vi "nanocal -- nuclear schottky fit -- 2x2 -- V9.vi"() -> ()   [LabVIEW 2021] (continued)
\"κ0\" -> 0.000000000000   ,  \"mm1\" -> 0.000000000000   ,  \"mm2\" -> 0.000000000000   ,  \"mm3\" -> 0.000000000000   ,  \"T\" -> 1.120000000000   ,  \"B\" -> 10.000000000000   ,  \"θ\" -> 0.000000000000   ,  \"Reoff\" -> 0.000000000000   ,  \"Imoff\" -> 0.000000000000   ,  \"στ1\" -> 0.000000000000   ,  \"στS\" -> 0.000000000000   ,  \"στN\" -> 0.000000000000    |>   , \n\"IDS0436_220527_RAW_cal__ref_\" ->   <|    \"ζ\" -> 0.020634042480   ,  \"τ1\" -> 0.020416898580   ,  \"τS\" -> 0.013006754143   ,  \"τN\" -> 0.000157221748   ,  \"τC\" -> 0.001868338850   ,  \"κ0\" -> 0.000000012250   ,  \"mm1\" -> 0.000033184482   ,  \"mm2\" -> 0.014698009084   ,  \"mm3\" -> 0.020989645793   ,  \"T\" -> 1.900000000000   ,  \"B\" -> 10.000000000000   ,  \"θ\" -> 0.000000000000   ,  \"Reoff\" -> -693877.551020413636   ,  \"Imoff\" -> 0.000000000000   ,  \"στ1\" -> 0.001009802597   ,  \"στS\" -> 0.000108538250   ,  \"στN\" -> 0.000005592624    |>   , \n\"IDS0436_220527_RAW_cal__sam_\" ->   <|    \"ζ\" -> 0.000000000000   ,  \"τ1\" -> 0.000000000000   ,  \"τS\" -> 0.000000000000   ,  \"τN\" -> 0.000000000000   ,  \"τC\" -> 0.000000000000   ,  \"κ0\" -> 0.000000000000   ,  \"mm1\" -> 0.000000000000   ,  \"mm2\" -> 0.000000000000   ,  \"mm3\" -> 0.000000000000   ,  \"T\" -> 1.900000000000   ,  \"B\" -> 10.000000000000   ,  \"θ\" -> 0.000000000000   ,  \"Reoff\" -> 0.000000000000   ,  \"Imoff\" -> 0.000000000000   ,  \"στ1\" -> 0.000000000000   ,  \"στS\" -> 0.000000000000   ,  \"στN\" -> 0.000000000000    |>   , \n\"IDS0437_220527_RAW_cal__ref_\" ->   <|    \"ζ\" -> 0.017700486500   ,  \"τ1\" -> 0.021195716861   ,  \"τS\" -> 0.009553240691   ,  \"τN\" -> 0.000096318625   ,  \"τC\" -> 0.001777778444   ,  \"κ0\" -> 0.000000022000   ,  \"mm1\" -> 0.000026199986   ,  \"mm2\" -> 0.011360732885   ,  \"mm3\" -> 0.021406923644   ,  \"T\" -> 3.100000000000   ,  \"B\" -> 10.000000000000   ,  \"θ\" -> 0.000000000000   ,  \"Reoff\" -> -326530.612244898453   ,  \"Imoff\" -> 0.000000000000   ,  \"στ1\" -> 0.003823035587   ,  \"στS\" -> 0.000080670014   ,  \"στN\" -> 0.000008312416    |>   , \n\"IDS0437_220527_RAW_cal__sam_\" ->   <|    \"ζ\" -> 0.000000000000   ,  \"τ1\" -> 0.000000000000   ,  \"τS\" -> 0.000000000000   ,  \"τN\" -> 0.000000000000   ,  \"τC\" -> 0.000000000000   ,  \"κ0\" -> 0.000000000000   ,  \"mm1\" -> 0.000000000000   ,  \"mm2\" -> 0.000000000000   ,  \"mm3\" -> 0.000000000000   ,  \"T\" -> 3.100000000000   ,  \"B\" -> 10.000000000000   ,  \"θ\" -> 0.000000000000   ,  \"Reoff\" -> 0.000000000000   ,  \"Imoff\" -> 0.000000000000   ,  \"στ1\" -> 0.000000000000   ,  \"στS\" -> 0.000000000000   ,  \"στN\" -> 0.000000000000    |>   , \n\"IDS0438_220527_RAW_cal__ref_\" ->   <|    \"ζ\" -> 0.017333863476   ,  \"τ1\" -> 0.021487771905   ,  \"τS\" -> 0.006060943357   ,  \"τN\" -> 0.000094743973   ,  \"τC\" -> 0.001680463551   ,  \"κ0\" -> 0.000000054800   ,  \"mm1\" -> 0.000022565233   ,  \"mm2\" -> 0.007769356044   ,  \"mm3\" -> 0.021638703353   ,  \"T\" -> 5.700000000000   ,  \"B\" -> 10.000000000000   ,  \"θ\" -> 0.000000000000   ,  \"Reoff\" -> -102040.816326530650   ,  \"Imoff\" -> 0.000000000000   ,  \"στ1\" -> 0.003634760564   ,  \"στS\" -> 0.000066823566   ,  \"στN\" -> 0.000004946508    |>   , \n\"IDS0438_220527_RAW_cal__sam_\" ->   <|    \"ζ\" -> 0.000000000000   ,  \"τ1\" -> 0.000000000000   ,  \"τS\" -> 0.000000000000   ,  \"τN\" -> 0.000000000000   ,  \"τC\" -> 0.000000000000   ,  \"κ0\" -> 0.000000000000   ,  \"mm1\" -> 0.000000000000   ,  \"mm2\" -> 0.000000000000   ,  \"mm3\" -> 0.000000000000   ,  \"T\" -> 5.700000000000   ,  \"B\" -> 10.000000000000   ,  \"θ\" -> 0.000000000000   ,  \"Reoff\" -> 0.000000000000   ,  \"Imoff\" -> 0.000000000000   ,  \"στ1\" -> 0.000000000000   ,  \"στS\" -> 0.000000000000   ,  \"στN\" -> 0.000000000000    |>   , \n\"IDS0439_220527_RAW_cal__ref_\" ->   <|    \"ζ\" -> 0.020515660719   ,  \"τ1\" -> 0.020182411708   ,  \"τS\" -> 0.016419895032   ,  \"τN\" -> 0.000240616919   ,  \"τC\" -> 0.002259910162   ,  \"κ0\" -> 0.000000008010   ,  \"mm1\" -> 0.000040116981   ,  \"mm2\" -> 0.017425178232   ,  \"mm3\" -> 0.021979340018   ,  \"T\" -> 1.280000000000   ,  \"B\" -> 10.000000000000   ,  \"θ\" -> 0.000000000000   ,  \"Reoff\" -> -693877.551020413636   ,  \"Imoff\" -> 0.000000000000   ,  \"στ1\" -> 0.001720696083   ,  \"στS\" -> 0.000105898596   ,  \"στN\" -> 0.000011441558    |>   , \n\"IDS0439_220527_RAW_cal__sam_\" ->   <|    \"ζ\" -> 0.000000000000   ,  \"τ1\" -> 0.000000000000   ,  \"τS\" -> 0.000000000000   ,  \"τN\" -> 0.000000000000   ,  \"τC\" -> 0.000000000000   ,  \"κ0\" -> 0.000000000000   ,  \"mm1\" -> 0.000000000000   ,  \"mm2\" -> 0.000000000000   ,  \"mm3\" -> 0.000000000000   ,  \"T\" -> 1.280000000000   ,  \"B\" -> 10.000000000000   ,  \"θ\" -> 0.000000000000   ,  \"Reoff\" -> 0.000000000000   ,  \"Imoff\" -> 0.000000000000   ,  \"στ1\" -> 0.000000000000   ,  \"στS\" -> 0.000000000000   ,  \"στN\" -> 0.000000000000    |>   , \n\"IDS0441_220527_RAW_cal__ref_\" ->   <|    \"ζ\" -> 0.245298177404   ,  \"τ1\" -> 0.085385227960   ,  \"τS\" -> 0.023089892303   ,  \"τN\" -> 0.011485885148   ,  \"τC\" -> 0.000787848696   ,  \"κ0\" -> 0.000000000810   ,  \"mm1\" -> 0.000151828666   ,  \"mm2\" -> 0.023847632864   ,  \"mm3\" -> 0.105230767769   ,  \"T\" -> 0.200000000000   ,  \"B\" -> 6.000000000000   ,  \"θ\" -> 0.000000000000   ,  \"Reoff\" -> -50367346.938775539400   ,  \"Imoff\" -> 0.000000000000   ,  \"στ1\" -> 0.073805144246   ,  \"στS\" -> 0.000832804395   ,  \"στN\" -> 0.007851231526    |>   , \n\"IDS0441_220527_RAW_cal__sam_\" ->   <|    \"ζ\" -> 0.000000000000   ,  \"τ1\" -> 0.000000000000   ,  \"τS\" -> 0.000000000000   ,  \"τN\" -> 0.000000000000   ,  \"τC\" -> 0.000000000000   ,  \"κ0\" -> 0.000000000000   ,  \"mm1\" -> 0.000000000000   ,  \"mm2\" -> 0.000000000000   ,  \"mm3\" -> 0.000000000000   ,  \"T\" -> 0.200000000000   ,  \"B\" -> 6.000000000000   ,  \"θ\" -> 0.000000000000   ,  \"Reoff\" -> 0.000000000000   ,  \"Imoff\" -> 0.000000000000   ,  \"στ1\" -> 0.000000000000   ,  \"στS\" -> 0.000000000000   ,  \"στN\" -> 0.000000000000    |>   , \n\"IDS0442_220528_RAW_cal__ref_\" ->   <|    \"ζ\" -> 0.649253803207   ,  \"τ1\" -> 0.189967266824   ,  \"τS\" -> 0.078891800944   ,  \"τN\" -> 0.111026532234   ,  \"τC\" -> 0.000810885423   ,  \"κ0\" -> 0.000000000435   ,  \"mm1\" -> 0.000318009867   ,  \"mm2\" -> 0.055339104870   ,  \"mm3\" -> 0.448344570802   ,  \"T\" -> 0.120000000000   ,  \"B\" -> 6.000000000000   ,  \"θ\" -> 0.000000000000   ,  \"Reoff\" -> -187755102.040816367000   ,  \"Imoff\" -> 0.000000000000   ,  \"στ1\" -> 0.116072095960   ,  \"στS\" -> 0.013830964310   ,  \"στN\" -> 0.055132667771    |>   , \n\"IDS0442_220528_RAW_cal__sam_\" ->   <|    \"ζ\" -> 0.000000000000   ,  \"τ1\" -> 0.000000000000   ,  \"τS\" -> 0.000000000000   ,  \"τN\" -> 0.000000000000   ,  \"τC\" -> 0.000000000000   ,  \"κ0\" -> 0.000000000000   ,  \"mm1\" -> 0.000000000000   ,  \"mm2\" -> 0.000000000000   ,  \"mm3\" -> 0.000000000000   ,  \"T\" -> 0.120000000000   ,  \"B\" -> 6.000000000000   ,  \"θ\" -> 0.000000000000   ,  \"Reoff\" -> 0.000000000000   ,  \"Imoff\" -> 0.000000000000   ,  \"στ1\" -> 0.000000000000   ,  \"στS\" -> 0.000000000000   ,  \"στN\" -> 0.000000000000    |>   , \n\"IDS0443_220528_RAW_cal__ref_\" ->   <|    \"ζ\" -> 0.445042406972   ,  \"τ1\" -> 0.128589504516   ,  \"τS\" -> 0.034654563108   ,  \"τN\" -> 0.043810211880   ,  \"τC\" -> 0.000810309510   ,  \"κ0\" -> 0.000000000605   ,  \"mm1\" -> 0.000246774346   ,  \"mm2\" -> 0.030747670130   ,  \"mm3\" -> 0.211790296861   ,  \"T\" -> 0.150000000000   ,  \"B\" -> 6.000000000000   ,  \"θ\" -> 0.000000000000   ,  \"Reoff\" -> -104489795.918367386000   ,  \"Imoff\" -> 0.000000000000   ,  \"στ1\" -> 0.161783937181   ,  \"στS\" -> 0.005303891089   ,  \"στN\" -> 0.043224722423    |>   , \n\"IDS0443_220528_RAW_cal__sam_\" ->   <|    \"ζ\" -> 0.000000000000   ,  \"τ1\" -> 0.000000000000   ,  \"τS\" -> 0.000000000000   ,  \"τN\" -> 0.000000000000   ,  \"τC\" -> 0.000000000000   ,  \"κ0\" -> 0.000000000000   ,  \"mm1\" -> 0.000000000000   ,  \"mm2\" -> 0.000000000000   ,  \"mm3\" -> 0.000000000000   ,  \"T\" -> 0.150000000000   ,  \"B\" -> 6.000000000000   ,  \"θ\" -> 0.000000000000   ,  \"Reoff\" -> 0.000000000000   ,  \"Imoff\" -> 0.000000000000   ,  \"στ1\" -> 0.000000000000   ,  \"στS\" -> 0.000000000000   ,  \"στN\" -> 0.000000000000    |>   , \n\"IDS0444_220528_RAW_cal__ref_\" ->   <|    \"ζ\" -> 0.346175274834   ,  \"τ1\" -> 0.111956082957   ,  \"τS\" -> 0.027343356843   ,  \"τN\" -> 0.025121384600   ,  \"τC\" -> 0.000749531065   ,  \"κ0\" -> 0.000000000740   ,  \"mm1\" -> 0.000189854194   ,  \"mm2\" -> 0.026751880765   ,  \"mm3\" -> 0.156390616794   ,  \"T\" -> 0.170000000000   ,  \"B\" -> 6.000000000000   ,  \"θ\" -> 0.000000000000   ,  \"Reoff\" -> -71183673.469387769700   ,  \"Imoff\" -> 0.000000000000   ,  \"στ1\" -> 0.050375037721   ,  \"στS\" -> 0.001079416051   ,  \"στN\" -> 0.009083705323    |>   , \n\"IDS0444_220528_RAW_cal__sam_\" ->   <|    \"ζ\" -> 0.000000000000   ,  \"τ1\" -> 0.000000000000   ,  \"τS\" -> 0.000000000000   ,  \"τN\" -> 0.000000000000   ,  \"τC\" -> 0.000000000000   ,  \"κ0\" -> 0.000000000000   ,  \"mm1\" -> 0.000000000000   ,  \"mm2\" -> 0.000000000000   ,  \"mm3\" -> 0.000000000000   ,  \"T\" -> 0.170000000000   ,  \"B\" -> 6.000000000000   ,  \"θ\" -> 0.000000000000   ,  \"Reoff\" -> 0.000000000000   ,  \"Imoff\" -> 0.000000000000   ,  \"στ1\" -> 0.000000000000   ,  \"στS\" -> 0.000000000000   ,  \"στN\" -> 0.000000000000    |>   , \n\"IDS0445_220528_RAW_cal__ref_\" ->   <|    \"ζ\" -> 0.167396769386   ,  \"τ1\" -> 0.076975995678   ,  \"τS\" -> 0.019126902976   ,  \"τN\" -> 0.005930151482   ,  \"τC\" -> 0.000960075113   ,  \"κ0\" -> 0.000000001240   ,  \"mm1\" -> 0.000132747039   ,  \"mm2\" -> 0.020623110398   ,  \"mm3\" -> 0.086431737778   ,  \"T\" -> 0.250000000000   ,  \"B\" -> 6.000000000000   ,  \"θ\" -> 0.000000000000   ,  \"Reoff\" -> -21224489.795918405100   ,  \"Imoff\" -> 0.000000000000   ,  \"στ1\" -> 0.058389287380   ,  \"στS\" -> 0.000426789295   ,  \"στN\" -> 0.003784929464    |>   , \n\"IDS0445_220528_RAW_cal__sam_\" ->   <|    \"ζ\" -> 0.000000000000   ,  \"τ1\" -> 0.000000000000   ,  \"τS\" -> 0.000000000000   ,  \"τN\" -> 0.000000000000   ,  \"τC\" -> 0.000000000000   ,  \"κ0\" -> 0.000000000000   ,  \"mm1\" -> 0.000000000000   ,  \"mm2\" -> 0.000000000000   ,  \"mm3\" -> 0.000000000000   ,  \"T\" -> 0.250000000000   ,  \"B\" -> 6.000000000000   ,  \"θ\" -> 0.000000000000   ,  \"Reoff\" -> 0.000000000000   ,  \"Imoff\" -> 0.000000000000   ,  \"στ1\" -> 0.000000000000   ,  \"στS\" -> 0.000000000000   ,  \"στN\" -> 0.000000000000    |>   , \n\"IDS0446_220528_RAW_cal__ref_\" ->   <|    \"ζ\" -> 0.116182318026   ,  \"τ1\" -> 0.081640310959   ,  \"τS\" -> 0.017704747394   ,  \"τN\" -> 0.003731217958   ,  \"τC\" -> 0.001140395347   ,  \"κ0\" -> 0.000000001560   ,  \"mm1\" -> 0.000112833833   ,  \"mm2\" -> 0.019484161721   ,  \"mm3\" -> 0.087110156248   ,  \"T\" -> 0.300000000000   ,  \"B\" -> 6.000000000000   ,  \"θ\" -> 0.000000000000   ,  \"Reoff\" -> -9836734.693877555430   ,  \"Imoff\" -> 0.000000000000   ,  \"στ1\" -> 0.008773282825   ,  \"στS\" -> 0.000191111466   ,  \"στN\" -> 0.000539753002    |>   , \n\"IDS0446_220528_RAW_cal__sam_\" ->   <|    \"ζ\" -> 0.000000000000   ,  \"τ1\" -> 0.000000000000   ,  \"τS\" -> 0.000000000000   ,  \"τN\" -> 0.000000000000   ,  \"τC\" -> 0.000000000000   ,  \"κ0\" -> 0.000000000000   ,  \"mm1\" -> 0.000000000000   ,  \"mm2\" -> 0.000000000000   ,  \"mm3\" -> 0.000000000000   ,  \"T\" -> 0.300000000000   ,  \"B\" -> 6.000000000000   ,  \"θ\" -> 0.000000000000   ,  \"Reoff\" -> 0.000000000000   ,  \"Imoff\" -> 0.000000000000   ,  \"στ1\" -> 0.000000000000   ,  \"στS\" -> 0.000000000000   ,  \"στN\" -> 0.000000000000    |>   , \n\"IDS0447_220528_RAW_cal__ref_\" ->   <|    \"ζ\" -> 0.082260507955   ,  \"τ1\" -> 0.097855412168   ,  \"τS\" -> 0.016892570352   ,  \"τN\" -> 0.002508450839   ,  \"τC\" -> 0.001377537548   ,  \"κ0\" -> 0.000000001980   ,  \"mm1\" -> 0.000097853534   ,  \"mm2\" -> 0.018911725587   ,  \"mm3\" -> 0.101220329644   ,  \"T\" -> 0.360000000000   ,  \"B\" -> 6.000000000000   ,  \"θ\" -> 0.000000000000   ,  \"Reoff\" -> -5918367.346938773990   ,  \"Imoff\" -> 0.000000000000   ,  \"στ1\" -> 0.011453835747   ,  \"στS\" -> 0.000169259584   ,  \"στN\" -> 0.000081203504    |>   , \n\"IDS0447_220528_RAW_cal__sam_\" ->   <|    \"ζ\" -> 0.000000000000   ,  \"τ1\" -> 0.000000000000   ,  \"τS\" -> 0.000000000000   ,  \"τN\" -> 0.000000000000   ,  \"τC\" -> 0.000000000000   ,  \"κ0\" -> 0.000000000000   ,  \"mm1\" -> 0.000000000000   ,  \"mm2\" -> 0.000000000000   ,  \"mm3\" -> 0.000000000000   ,  \"T\" -> 0.360000000000   ,  \"B\" -> 6.000000000000   ,  \"θ\" -> 0.000000000000   ,  \"Reoff\" -> 0.000000000000   ,  \"Imoff\" -> 0.000000000000   ,  \"στ1\" -> 0.000000000000   ,  \"στS\" -> 0.000000000000   ,  \"στN\" -> 0.000000000000    |>   , \n\"IDS0448_220528_RAW_cal__ref_\" ->   <|    \"ζ\" -> 0.062921401678   ,  \"τ1\" -> 0.104858235464   ,  \"τS\" -> 0.016995205436   ,  \"τN\" -> 0.001995569768   ,  \"τC\" -> 0.001676394953   ,  \"κ0\" -> 0.000000002390   ,  \"mm1\" -> 0.000091230686   ,  \"mm2\" -> 0.019175235813   ,  \"mm3\" -> 0.107453865317   ,  \"T\" -> 0.420000000000   ,  \"B\" -> 6.000000000000   ,  \"θ\" -> 0.000000000000   ,  \"Reoff\" -> -3224489.795918367800   ,  \"Imoff\" -> 0.000000000000   ,  \"στ1\" -> 0.006534185660   ,  \"στS\" -> 0.000117840372   ,  \"στN\" -> 0.000044604880    |>   , \n\"IDS0448_220528_RAW_cal__sam_\" ->   <|    \"ζ\" -> 0.000000000000   ,  \"τ1\" -> 0.000000000000   ,  \"τS\" -> 0.000000000000   ,  \"τN\" -> 0.000000000000   ,  \"τC\" -> 0.000000000000   ,  \"κ0\" -> 0.000000000000   ,  \"mm1\" -> 0.000000000000   ,  \"mm2\" -> 0.000000000000   ,  \"mm3\" -> 0.000000000000   ,  \"T\" -> 0.420000000000   ,  \"B\" -> 6.000000000000   ,  \"θ\" -> 0.000000000000   ,  \"Reoff\" -> 0.000000000000   ,  \"Imoff\" -> 0.000000000000   ,  \"στ1\" -> 0.000000000000   ,  \"στS\" -> 0.000000000000   ,  \"στN\" -> 0.000000000000    |>   , \n\"IDS0449_220528_RAW_cal__ref_\" ->   <|    \"ζ\" -> 0.047884623717   ,  \"τ1\" -> 0.131080457695   ,  \"τS\" -> 0.018007411450   ,  \"τN\" -> 0.000981367223   ,  \"τC\" -> 0.001725529599   ,  \"κ0\" -> 0.000000003050   ,  \"mm1\" -> 0.000072499299   ,  \"mm2\" -> 0.020333963628   ,  \"mm3\" -> 0.132297573561   ,  \"T\" -> 0.520000000000   ,  \"B\" -> 6.000000000000   ,  \"θ\" -> 0.000000000000   ,  \"Reoff\" -> -2734693.877551019190   ,  \"Imoff\" -> 0.000000000000   ,  \"στ1\" -> 0.004608574933   ,  \"στS\" -> 0.000117579650   ,  \"στN\" -> 0.000012752595    |>   , \n\"IDS0449_220528_RAW_cal__sam_\" ->   <|    \"ζ\" -> 0.000000000000   ,  \"τ1\" -> 0.000000000000   ,  \"τS\" -> 0.000000000000   ,  \"τN\" -> 0.000000000000   ,  \"τC\" -> 0.000000000000   ,  \"κ0\" -> 0.000000000000   ,  \"mm1\" -> 0.000000000000   ,  \"mm2\" -> 0.000000000000   ,  \"mm3\" -> 0.000000000000   ,  \"T\" -> 0.520000000000   ,  \"B\" -> 6.000000000000   ,  \"θ\" -> 0.000000000000   ,  \"Reoff\" -> 0.000000000000   ,  \"Imoff\" -> 0.000000000000   ,  \"στ1\" -> 0.000000000000   ,  \"στS\" -> 0.000000000000   ,  \"στN\" -> 0.000000000000    |>   , \n\"IDS0450_220528_RAW_cal__ref_\" ->   <|    \"ζ\" -> 0.039229464810   ,  \"τ1\" -> 0.132250871958   ,  \"τS\" -> 0.019567524350   ,  \"τN\" -> 0.000645572028   ,  \"τC\" -> 0.002216107396   ,  \"κ0\" -> 0.000000003710   ,  \"mm1\" -> 0.000075688104   ,  \"mm2\" -> 0.022339257593   ,  \"mm3\" -> 0.133058078988   ,  \"T\" -> 0.620000000000   ,  \"B\" -> 6.000000000000   ,  \"θ\" -> 0.000000000000   ,  \"Reoff\" -> -1836734.693877549840   ,  \"Imoff\" -> 0.000000000000   ,  \"στ1\" -> 0.013891983729   ,  \"στS\" -> 0.000275228505   ,  \"στN\" -> 0.000014669309    |>   , \n\"IDS0450_220528_RAW_cal__sam_\" ->   <|    \"ζ\" -> 0.000000000000   ,  \"τ1\" -> 0.000000000000   ,  \"τS\" -> 0.000000000000   ,  \"τN\" -> 0.000000000000   ,  \"τC\" -> 0.000000000000   ,  \"κ0\" -> 0.000000000000   ,  \"mm1\" -> 0.000000000000   ,  \"mm2\" -> 0.000000000000   ,  \"mm3\" -> 0.000000000000   ,  \"T\" -> 0.620000000000   ,  \"B\" -> 6.000000000000   ,  \"θ\" -> 0.000000000000   ,  \"Reoff\" -> 0.000000000000   ,  \"Imoff\" -> 0.000000000000   ,  \"στ1\" -> 0.000000000000   ,  \"στS\" -> 0.000000000000   ,  \"στN\" -> 0.000000000000    |>   , \n\"IDS0451_220528_RAW_cal__ref_\" ->   <|    \"ζ\" -> 0.026807399567   ,  \"τ1\" -> 0.154252177981   ,  \"τS\" -> 0.023590031432   ,  \"τN\" -> 0.000319958180   ,  \"τC\" -> 0.003023021175   ,  \"κ0\" -> 0.000000005180   ,  \"mm1\" -> 0.000070348215   ,  \"mm2\" -> 0.027105077142   ,  \"mm3\" -> 0.154650728056   ,  \"T\" -> 0.820000000000   ,  \"B\" -> 6.000000000000   ,  \"θ\" -> 0.000000000000   ,  \"Reoff\" -> -612244.897959182038   ,  \"Imoff\" -> 0.000000000000   ,  \"στ1\" -> 0.012428803494   ,  \"στS\" -> 0.000182806750   ,  \"στN\" -> 0.000002712737    |>   , \n\"IDS0451_220528_RAW_cal__sam_\" ->   <|    \"ζ\" -> 0.000000000000   ,  \"τ1\" -> 0.000000000000   ,  \"τS\" -> 0.000000000000   ,  \"τN\" -> 0.000000000000   ,  \"τC\" -> 0.000000000000   ,  \"κ0\" -> 0.000000000000   ,  \"mm1\" -> 0.000000000000   ,  \"mm2\" -> 0.000000000000   ,  \"mm3\" -> 0.000000000000   ,  \"T\" -> 0.820000000000   ,  \"B\" -> 6.000000000000   ,  \"θ\" -> 0.000000000000   ,  \"Reoff\" -> 0.000000000000   ,  \"Imoff\" -> 0.000000000000   ,  \"στ1\" -> 0.000000000000   ,  \"στS\" -> 0.000000000000   ,  \"στN\" -> 0.000000000000    |>   , \n\"IDS0452_220528_RAW_cal__ref_\" ->   <|    \"ζ\" -> 0.022314359927   ,  \"τ1\" -> 0.160926117275   ,  \"τS\" -> 0.032134640679   ,  \"τN\" -> 0.000145739971   ,  \"τC\" -> 0.002824145065   ,  \"κ0\" -> 0.000000007200   ,  \"mm1\" -> 0.000056854280   ,  \"mm2\" -> 0.035576714114   ,  \"mm3\" -> 0.161117390629   ,  \"T\" -> 1.120000000000   ,  \"B\" -> 6.000000000000   ,  \"θ\" -> 0.000000000000   ,  \"Reoff\" -> -702040.816326530649   ,  \"Imoff\" -> 0.000000000000   ,  \"στ1\" -> 0.054678579319   ,  \"στS\" -> 0.000310139427   ,  \"στN\" -> 0.000011071963    |>   , \n\"IDS0452_220528_RAW_cal__sam_\" ->   <|    \"ζ\" -> 0.000000000000   ,  \"τ1\" -> 0.000000000000   ,  \"τS\" -> 0.000000000000   ,  \"τN\" -> 0.000000000000   ,  \"τC\" -> 0.000000000000   ,  \"κ0\" -> 0.000000000000   ,  \"mm1\" -> 0.000000000000   ,  \"mm2\" -> 0.000000000000   ,  \"mm3\" -> 0.000000000000   ,  \"T\" -> 1.120000000000   ,  \"B\" -> 6.000000000000   ,  \"θ\" -> 0.000000000000   ,  \"Reoff\" -> 0.000000000000   ,  \"Imoff\" -> 0.000000000000   ,  \"στ1\" -> 0.000000000000   ,  \"στS\" -> 0.000000000000   ,  \"στN\" -> 0.000000000000    |>   , \n\"IDS0453_220529_RAW_cal__ref_\" ->   <|    \"ζ\" -> 0.018679261222   ,  \"τ1\" -> 0.150357444962   ,  \"τS\" -> 0.034780809519   ,  \"τN\" -> 0.000073406760   ,  \"τC\" -> 0.002819029609   ,  \"κ0\" -> 0.000000011200   ,  \"mm1\" -> 0.000047942172   ,  \"mm2\" -> 0.038176131794   ,  \"mm3\" -> 0.150457667894   ,  \"T\" -> 1.700000000000   ,  \"B\" -> 6.000000000000   ,  \"θ\" -> 0.000000000000   ,  \"Reoff\" -> -297959.183673469349   ,  \"Imoff\" -> 0.000000000000   ,  \"στ1\" -> 0.025512305357   ,  \"στS\" -> 0.000555960803   ,  \"στN\" -> 0.000005395580    |>   , \n\"IDS0453_220529_RAW_cal__sam_\" ->   <|    \"ζ\" -> 0.000000000000   ,  \"τ1\" -> 0.000000000000   ,  \"τS\" -> 0.000000000000   ,  \"τN\" -> 0.000000000000   ,  \"τC\" -> 0.000000000000   ,  \"κ0\" -> 0.000000000000   ,  \"mm1\" -> 0.000000000000   ,  \"mm2\" -> 0.000000000000   ,  \"mm3\" -> 0.000000000000   ,  \"T\" -> 1.700000000000   ,  \"B\" -> 6.000000000000   ,  \"θ\" -> 0.000000000000   ,  \"Reoff\" -> 0.000000000000   ,  \"Imoff\" -> 0.000000000000   ,  \"στ1\" -> 0.000000000000   ,  \"στS\" -> 0.000000000000   ,  \"στN\" -> 0.000000000000    |>   , \n\"IDS0454_220529_RAW_cal__ref_\" ->   <|    \"ζ\" -> 0.017513842872   ,  \"τ1\" -> 0.023424290493   ,  \"τS\" -> 0.014683078864   ,  \"τN\" -> 0.000047379208   ,  \"τC\" -> 0.003106112976   ,  \"κ0\" -> 0.000000012600   ,  \"mm1\" -> 0.000044370583   ,  \"mm2\" -> 0.017847763479   ,  \"mm3\" -> 0.023626714407   ,  \"T\" -> 1.900000000000   ,  \"B\" -> 6.000000000000   ,  \"θ\" -> 0.000000000000   ,  \"Reoff\" -> -371428.571428571827   ,  \"Imoff\" -> 0.000000000000   ,  \"στ1\" -> 0.007486573720   ,  \"στS\" -> 0.000328189496   ,  \"στN\" -> 0.000005492338    |>   , \n\"IDS0454_220529_RAW_cal__sam_\" ->   <|    \"ζ\" -> 0.000000000000   ,  \"τ1\" -> 0.000000000000   ,  \"τS\" -> 0.000000000000   ,  \"τN\" -> 0.000000000000   ,  \"τC\" -> 0.000000000000   ,  \"κ0\" -> 0.000000000000   ,  \"mm1\" -> 0.000000000000   ,  \"mm2\" -> 0.000000000000   ,  \"mm3\" -> 0.000000000000   ,  \"T\" -> 1.900000000000   ,  \"B\" -> 6.000000000000   ,  \"θ\" -> 0.000000000000   ,  \"Reoff\" -> 0.000000000000   ,  \"Imoff\" -> 0.000000000000   ,  \"στ1\" -> 0.000000000000   ,  \"στS\" -> 0.000000000000   ,  \"στN\" -> 0.000000000000    |>   , \n\"IDS0455_220529_RAW_cal__ref_\" ->   <|    \"ζ\" -> 0.017684542475   ,  \"τ1\" -> 0.025415252258   ,  \"τS\" -> 0.009236528363   ,  \"τN\" -> 0.000017905293   ,  \"τC\" -> 0.002401600721   ,  \"κ0\" -> 0.000000022300   ,  \"mm1\" -> 0.000033334613   ,  \"mm2\" -> 0.011752475280   ,  \"mm3\" -> 0.025449137167   ,  \"T\" -> 3.100000000000   ,  \"B\" -> 6.000000000000   ,  \"θ\" -> 0.000000000000   ,  \"Reoff\" -> -224489.795918366871   ,  \"Imoff\" -> 0.000000000000   ,  \"στ1\" -> 0.002319336344   ,  \"στS\" -> 0.000088789026   ,  \"στN\" -> 0.000000711840    |>   , \n\"IDS0455_220529_RAW_cal__sam_\" ->   <|    \"ζ\" -> 0.000000000000   ,  \"τ1\" -> 0.000000000000   ,  \"τS\" -> 0.000000000000   ,  \"τN\" -> 0.000000000000   ,  \"τC\" -> 0.000000000000   ,  \"κ0\" -> 0.000000000000   ,  \"mm1\" -> 0.000000000000   ,  \"mm2\" -> 0.000000000000   ,  \"mm3\" -> 0.000000000000   ,  \"T\" -> 3.100000000000   ,  \"B\" -> 6.000000000000   ,  \"θ\" -> 0.000000000000   ,  \"Reoff\" -> 0.000000000000   ,  \"Imoff\" -> 0.000000000000   ,  \"στ1\" -> 0.000000000000   ,  \"στS\" -> 0.000000000000   ,  \"στN\" -> 0.000000000000    |>   , \n\"IDS0456_220529_RAW_cal__ref_\" ->   <|    \"ζ\" -> 0.018735255997   ,  \"τ1\" -> 0.025807065758   ,  \"τS\" -> 0.005944253757   ,  \"τN\" -> 0.000004775198   ,  \"τC\" -> 0.001961268842   ,  \"κ0\" -> 0.000000054800   ,  \"mm1\" -> 0.000027338307   ,  \"mm2\" -> 0.007987373292   ,  \"mm3\" -> 0.025814108537   ,  \"T\" -> 5.700000000000   ,  \"B\" -> 6.000000000000   ,  \"θ\" -> 0.000000000000   ,  \"Reoff\" -> -77551.020408162847   ,  \"Imoff\" -> 0.000000000000   ,  \"στ1\" -> 0.003676288803   ,  \"στS\" -> 0.001284267534   ,  \"στN\" -> 0.000002465031    |>   , \n\"IDS0456_220529_RAW_cal__sam_\" ->   <|    \"ζ\" -> 0.000000000000   ,  \"τ1\" -> 0.000000000000   ,  \"τS\" -> 0.000000000000   ,  \"τN\" -> 0.000000000000   ,  \"τC\" -> 0.000000000000   ,  \"κ0\" -> 0.000000000000   ,  \"mm1\" -> 0.000000000000   ,  \"mm2\" -> 0.000000000000   ,  \"mm3\" -> 0.000000000000   ,  \"T\" -> 5.700000000000   ,  \"B\" -> 6.000000000000   ,  \"θ\" -> 0.000000000000   ,  \"Reoff\" -> 0.000000000000   ,  \"Imoff\" -> 0.000000000000   ,  \"στ1\" -> 0.000000000000   ,  \"στS\" -> 0.000000000000   ,  \"στN\" -> 0.000000000000    |>   , \n\"IDS0458_220529_RAW_cal__ref_\" ->   <|    \"ζ\" -> 0.271949590763   ,  \"τ1\" -> 0.082491161116   ,  \"τS\" -> 0.016634017124   ,  \"τN\" -> 0.004711774467   ,  \"τC\" -> 0.000759404494   ,  \"κ0\" -> 0.000000000880   ,  \"mm1\" -> 0.000157873787   ,  \"mm2\" -> 0.019859290085   ,  \"mm3\" -> 0.090384172617   ,  \"T\" -> 0.200000000000   ,  \"B\" -> 4.000000000000   ,  \"θ\" -> 0.000000000000   ,  \"Reoff\" -> -53755102.040816329400   ,  \"Imoff\" -> 0.000000000000   ,  \"στ1\" -> 0.009172162575   ,  \"στS\" -> 0.000087849728   ,  \"στN\" -> 0.000215184537    |>   , \n\"IDS0458_220529_RAW_cal__sam_\" ->   <|    \"ζ\" -> 0.000000000000   ,  \"τ1\" -> 0.000000000000   ,  \"τS\" -> 0.000000000000   ,  \"τN\" -> 0.000000000000   ,  \"τC\" -> 0.000000000000   ,  \"κ0\" -> 0.000000000000   ,  \"mm1\" -> 0.000000000000   ,  \"mm2\" -> 0.000000000000   ,  \"mm3\" -> 0.000000000000   ,  \"T\" -> 0.200000000000   ,  \"B\" -> 4.000000000000   ,  \"θ\" -> 0.000000000000   ,  \"Reoff\" -> 0.000000000000   ,  \"Imoff\" -> 0.000000000000   ,  \"στ1\" -> 0.000000000000   ,  \"στS\" -> 0.000000000000   ,  \"στN\" -> 0.000000000000    |>   , \n\"IDS0459_220529_RAW_cal__ref_\" ->   <|    \"ζ\" -> 0.169028221284   ,  \"τ1\" -> 0.092219125546   ,  \"τS\" -> 0.014617231308   ,  \"τN\" -> 0.003004665048   ,  \"τC\" -> 0.000894699791   ,  \"κ0\" -> 0.000000001215   ,  \"mm1\" -> 0.000123777676   ,  \"mm2\" -> 0.017061745572   ,  \"mm3\" -> 0.096528796242   ,  \"T\" -> 0.250000000000   ,  \"B\" -> 4.000000000000   ,  \"θ\" -> 0.000000000000   ,  \"Reoff\" -> -23428571.428571432800   ,  \"Imoff\" -> 0.000000000000   ,  \"στ1\" -> 0.009019898069   ,  \"στS\" -> 0.000072357815   ,  \"στN\" -> 0.000072194130    |>   , \n\"IDS0459_220529_RAW_cal__sam_\" ->   <|    \"ζ\" -> 0.000000000000   ,  \"τ1\" -> 0.000000000000   ,  \"τS\" -> 0.000000000000   ,  \"τN\" -> 0.000000000000   ,  \"τC\" -> 0.000000000000   ,  \"κ0\" -> 0.000000000000   ,  \"mm1\" -> 0.000000000000   ,  \"mm2\" -> 0.000000000000   ,  \"mm3\" -> 0.000000000000   ,  \"T\" -> 0.250000000000   ,  \"B\" -> 4.000000000000   ,  \"θ\" -> 0.000000000000   ,  \"Reoff\" -> 0.000000000000   ,  \"Imoff\" -> 0.000000000000   ,  \"στ1\" -> 0.000000000000   ,  \"στS\" -> 0.000000000000   ,  \"στN\" -> 0.000000000000    |>   , \n\"IDS0460_220529_RAW_cal__ref_\" ->   <|    \"ζ\" -> 0.121095025204   ,  \"τ1\" -> 0.101406294737   ,  \"τS\" -> 0.013797908139   ,  \"τN\" -> 0.002167085296   ,  \"τC\" -> 0.000940421698   ,  \"κ0\" -> 0.000000001550   ,  \"mm1\" -> 0.000096322687   ,  \"mm2\" -> 0.015862507367   ,  \"mm3\" -> 0.104286161098   ,  \"T\" -> 0.300000000000   ,  \"B\" -> 4.000000000000   ,  \"θ\" -> 0.000000000000   ,  \"Reoff\" -> -14857142.857142865700   ,  \"Imoff\" -> 0.000000000000   ,  \"στ1\" -> 0.003344660593   ,  \"στS\" -> 0.000083531617   ,  \"στN\" -> 0.000031930335    |>   , \n\"IDS0460_220529_RAW_cal__sam_\" ->   <|    \"ζ\" -> 0.000000000000   ,  \"τ1\" -> 0.000000000000   ,  \"τS\" -> 0.000000000000   ,  \"τN\" -> 0.000000000000   ,  \"τC\" -> 0.000000000000   ,  \"κ0\" -> 0.000000000000   ,  \"mm1\" -> 0.000000000000   ,  \"mm2\" -> 0.000000000000   ,  \"mm3\" -> 0.000000000000   ,  \"T\" -> 0.300000000000   ,  \"B\" -> 4.000000000000   ,  \"θ\" -> 0.000000000000   ,  \"Reoff\" -> 0.000000000000   ,  \"Imoff\" -> 0.000000000000   ,  \"στ1\" -> 0.000000000000   ,  \"στS\" -> 0.000000000000   ,  \"στN\" -> 0.000000000000    |>   , \n\"IDS0461_220529_RAW_cal__ref_\" ->   <|    \"ζ\" -> 0.088720032208   ,  \"τ1\" -> 0.108699367297   ,  \"τS\" -> 0.013278602208   ,  \"τN\" -> 0.001545664659   ,  \"τC\" -> 0.001067836739   ,  \"κ0\" -> 0.000000001950   ,  \"mm1\" -> 0.000081459775   ,  \"mm2\" -> 0.015170211659   ,  \"mm3\" -> 0.110655008903   ,  \"T\" -> 0.360000000000   ,  \"B\" -> 4.000000000000   ,  \"θ\" -> 0.000000000000   ,  \"Reoff\" -> -9714285.714285701520   ,  \"Imoff\" -> 0.000000000000   ,  \"στ1\" -> 0.011282789082   ,  \"στS\" -> 0.000097113540   ,  \"στN\" -> 0.000042096921    |>   , \n\"IDS0461_220529_RAW_cal__sam_\" ->   <|    \"ζ\" -> 0.000000000000   ,  \"τ1\" -> 0.000000000000   ,  \"τS\" -> 0.000000000000   ,  \"τN\" -> 0.000000000000   ,  \"τC\" -> 0.000000000000   ,  \"κ0\" -> 0.000000000000   ,  \"mm1\" -> 0.000000000000   ,  \"mm2\" -> 0.000000000000   ,  \"mm3\" -> 0.000000000000   ,  \"T\" -> 0.360000000000   ,  \"B\" -> 4.000000000000   ,  \"θ\" -> 0.000000000000   ,  \"Reoff\" -> 0.000000000000   ,  \"Imoff\" -> 0.000000000000   ,  \"στ1\" -> 0.000000000000   ,  \"στS\" -> 0.000000000000   ,  \"στN\" -> 0.000000000000    |>   , \n\"IDS0462_220530_RAW_cal__ref_\" ->   <|    \"ζ\" -> 0.343667501463   ,  \"τ1\" -> 0.112483041616   ,  \"τS\" -> 0.019628128809   ,  \"τN\" -> 0.010154591080   ,  \"τC\" -> 0.000829297605   ,  \"κ0\" -> 0.000000000715   ,  \"mm1\" -> 0.000207215692   ,  \"mm2\" -> 0.023410434838   ,  \"mm3\" -> 0.129712761510   ,  \"T\" -> 0.170000000000   ,  \"B\" -> 4.000000000000   ,  \"θ\" -> 0.000000000000   ,  \"Reoff\" -> -62857142.857142865700   ,  \"Imoff\" -> 0.000000000000   ,  \"στ1\" -> 0.089687632936   ,  \"στS\" -> 0.000139405002   ,  \"στN\" -> 0.005363489281    |>   , \n\"IDS0462_220530_RAW_cal__sam_\" ->   <|    \"ζ\" -> 0.000000000000   ,  \"τ1\" -> 0.000000000000   ,  \"τS\" -> 0.000000000000   ,  \"τN\" -> 0.000000000000   ,  \"τC\" -> 0.000000000000   ,  \"κ0\" -> 0.000000000000   ,  \"mm1\" -> 0.000000000000   ,  \"mm2\" -> 0.000000000000   ,  \"mm3\" -> 0.000000000000   ,  \"T\" -> 0.170000000000   ,  \"B\" -> 4.000000000000   ,  \"θ\" -> 0.000000000000   ,  \"Reoff\" -> 0.000000000000   ,  \"Imoff\" -> 0.000000000000   ,  \"στ1\" -> 0.000000000000   ,  \"στS\" -> 0.000000000000   ,  \"στN\" -> 0.000000000000    |>   , \n\"IDS0463_220530_RAW_cal__ref_\" ->   <|    \"ζ\" -> 0.430227807451   ,  \"τ1\" -> 0.103641258629   ,  \"τS\" -> 0.021841444015   ,  \"τN\" -> 0.013133276363   ,  \"τC\" -> 0.000817797243   ,  \"κ0\" -> 0.000000000620   ,  \"mm1\" -> 0.000241540150   ,  \"mm2\" -> 0.025640890482   ,  \"mm3\" -> 0.128598442882   ,  \"T\" -> 0.150000000000   ,  \"B\" -> 4.000000000000   ,  \"θ\" -> 0.000000000000   ,  \"Reoff\" -> -76204081.632653057600   ,  \"Imoff\" -> 0.000000000000   ,  \"στ1\" -> 0.056966109308   ,  \"στS\" -> 0.000433843322   ,  \"στN\" -> 0.005482906809    |>   , \n\"IDS0463_220530_RAW_cal__sam_\" ->   <|    \"ζ\" -> 0.000000000000   ,  \"τ1\" -> 0.000000000000   ,  \"τS\" -> 0.000000000000   ,  \"τN\" -> 0.000000000000   ,  \"τC\" -> 0.000000000000   ,  \"κ0\" -> 0.000000000000   ,  \"mm1\" -> 0.000000000000   ,  \"mm2\" -> 0.000000000000   ,  \"mm3\" -> 0.000000000000   ,  \"T\" -> 0.150000000000   ,  \"B\" -> 4.000000000000   ,  \"θ\" -> 0.000000000000   ,  \"Reoff\" -> 0.000000000000   ,  \"Imoff\" -> 0.000000000000   ,  \"στ1\" -> 0.000000000000   ,  \"στS\" -> 0.000000000000   ,  \"στN\" -> 0.000000000000    |>   , \n\"IDS0464_220530_RAW_cal__ref_\" ->   <|    \"ζ\" -> 0.675671528717   ,  \"τ1\" -> 0.134361338288   ,  \"τS\" -> 0.029407446025   ,  \"τN\" -> 0.029781674231   ,  \"τC\" -> 0.000802871531   ,  \"κ0\" -> 0.000000000450   ,  \"mm1\" -> 0.000320592060   ,  \"mm2\" -> 0.033310531198   ,  \"mm3\" -> 0.200714610183   ,  \"T\" -> 0.120000000000   ,  \"B\" -> 4.000000000000   ,  \"θ\" -> 0.000000000000   ,  \"Reoff\" -> -173428571.428571433000   ,  \"Imoff\" -> 0.000000000000   ,  \"στ1\" -> 0.117118369535   ,  \"στS\" -> 0.002310482505   ,  \"στN\" -> 0.019921704088    |>   , \n\"IDS0464_220530_RAW_cal__sam_\" ->   <|    \"ζ\" -> 0.000000000000   ,  \"τ1\" -> 0.000000000000   ,  \"τS\" -> 0.000000000000   ,  \"τN\" -> 0.000000000000   ,  \"τC\" -> 0.000000000000   ,  \"κ0\" -> 0.000000000000   ,  \"mm1\" -> 0.000000000000   ,  \"mm2\" -> 0.000000000000   ,  \"mm3\" -> 0.000000000000   ,  \"T\" -> 0.120000000000   ,  \"B\" -> 4.000000000000   ,  \"θ\" -> 0.000000000000   ,  \"Reoff\" -> 0.000000000000   ,  \"Imoff\" -> 0.000000000000   ,  \"στ1\" -> 0.000000000000   ,  \"στS\" -> 0.000000000000   ,  \"στN\" -> 0.000000000000    |>   , \n\"IDS0465_220530_RAW_cal__ref_\" ->   <|    \"ζ\" -> 0.065985765394   ,  \"τ1\" -> 0.113805435970   ,  \"τS\" -> 0.013450011184   ,  \"τN\" -> 0.001342731867   ,  \"τC\" -> 0.001243319385   ,  \"κ0\" -> 0.000000002410   ,  \"mm1\" -> 0.000071145975   ,  \"mm2\" -> 0.015287668803   ,  \"mm3\" -> 0.115458794101   ,  \"T\" -> 0.430000000000   ,  \"B\" -> 4.000000000000   ,  \"θ\" -> 0.000000000000   ,  \"Reoff\" -> -5918367.346938773990   ,  \"Imoff\" -> 0.000000000000   ,  \"στ1\" -> 0.012030942275   ,  \"στS\" -> 0.000092415308   ,  \"στN\" -> 0.000055296571    |>   , \n\"IDS0465_220530_RAW_cal__sam_\" ->   <|    \"ζ\" -> 0.000000000000   ,  \"τ1\" -> 0.000000000000   ,  \"τS\" -> 0.000000000000   ,  \"τN\" -> 0.000000000000   ,  \"τC\" -> 0.000000000000   ,  \"κ0\" -> 0.000000000000   ,  \"mm1\" -> 0.000000000000   ,  \"mm2\" -> 0.000000000000   ,  \"mm3\" -> 0.000000000000   ,  \"T\" -> 0.430000000000   ,  \"B\" -> 4.000000000000   ,  \"θ\" -> 0.000000000000   ,  \"Reoff\" -> 0.000000000000   ,  \"Imoff\" -> 0.000000000000   ,  \"στ1\" -> 0.000000000000   ,  \"στS\" -> 0.000000000000   ,  \"στN\" -> 0.000000000000    |>   , \n\"IDS0466_220530_RAW_cal__ref_\" ->   <|    \"ζ\" -> 0.050274873948   ,  \"τ1\" -> 0.117572813394   ,  \"τS\" -> 0.013965174353   ,  \"τN\" -> 0.000622498353   ,  \"τC\" -> 0.001752185729   ,  \"κ0\" -> 0.000000003045   ,  \"mm1\" -> 0.000075268427   ,  \"mm2\" -> 0.016239468880   ,  \"mm3\" -> 0.118331327928   ,  \"T\" -> 0.530000000000   ,  \"B\" -> 4.000000000000   ,  \"θ\" -> 0.000000000000   ,  \"Reoff\" -> -3204081.632653061300   ,  \"Imoff\" -> 0.000000000000   ,  \"στ1\" -> 0.009611649331   ,  \"στS\" -> 0.000172547734   ,  \"στN\" -> 0.000019241473    |>   , \n\"IDS0466_220530_RAW_cal__sam_\" ->   <|    \"ζ\" -> 0.000000000000   ,  \"τ1\" -> 0.000000000000   ,  \"τS\" -> 0.000000000000   ,  \"τN\" -> 0.000000000000   ,  \"τC\" -> 0.000000000000   ,  \"κ0\" -> 0.000000000000   ,  \"mm1\" -> 0.000000000000   ,  \"mm2\" -> 0.000000000000   ,  \"mm3\" -> 0.000000000000   ,  \"T\" -> 0.530000000000   ,  \"B\" -> 4.000000000000   ,  \"θ\" -> 0.000000000000   ,  \"Reoff\" -> 0.000000000000   ,  \"Imoff\" -> 0.000000000000   ,  \"στ1\" -> 0.000000000000   ,  \"στS\" -> 0.000000000000   ,  \"στN\" -> 0.000000000000    |>   , \n\"IDS0467_220530_RAW_cal__ref_\" ->   <|    \"ζ\" -> 0.041054990767   ,  \"τ1\" -> 0.119173098156   ,  \"τS\" -> 0.015405145420   ,  \"τN\" -> 0.000278319894   ,  \"τC\" -> 0.001789500233   ,  \"κ0\" -> 0.000000003708   ,  \"mm1\" -> 0.000063714353   ,  \"mm2\" -> 0.017712825393   ,  \"mm3\" -> 0.119513408481   ,  \"T\" -> 0.620000000000   ,  \"B\" -> 4.000000000000   ,  \"θ\" -> 0.000000000000   ,  \"Reoff\" -> -2755102.040816326160   ,  \"Imoff\" -> 0.000000000000   ,  \"στ1\" -> 0.018149556060   ,  \"στS\" -> 0.000211563346   ,  \"στN\" -> 0.000013374065    |>   , \n\"IDS0467_220530_RAW_cal__sam_\" ->   <|    \"ζ\" -> 0.000000000000   ,  \"τ1\" -> 0.000000000000   ,  \"τS\" -> 0.000000000000   ,  \"τN\" -> 0.000000000000   ,  \"τC\" -> 0.000000000000   ,  \"κ0\" -> 0.000000000000   ,  \"mm1\" -> 0.000000000000   ,  \"mm2\" -> 0.000000000000   ,  \"mm3\" -> 0.000000000000   ,  \"T\" -> 0.620000000000   ,  \"B\" -> 4.000000000000   ,  \"θ\" -> 0.000000000000   ,  \"Reoff\" -> 0.000000000000   ,  \"Imoff\" -> 0.000000000000   ,  \"στ1\" -> 0.000000000000   ,  \"στS\" -> 0.000000000000   ,  \"στN\" -> 0.000000000000    |>   , \n\"IDS0468_220530_RAW_cal__ref_\" ->   <|    \"ζ\" -> 0.028502781656   ,  \"τ1\" -> 0.123145264277   ,  \"τS\" -> 0.019280232525   ,  \"τN\" -> 0.000154237911   ,  \"τC\" -> 0.002123664207   ,  \"κ0\" -> 0.000000005085   ,  \"mm1\" -> 0.000053289074   ,  \"mm2\" -> 0.021865908006   ,  \"mm3\" -> 0.123338138308   ,  \"T\" -> 0.820000000000   ,  \"B\" -> 4.000000000000   ,  \"θ\" -> 0.000000000000   ,  \"Reoff\" -> -1265306.122448980810   ,  \"Imoff\" -> 0.000000000000   ,  \"στ1\" -> 0.018340702428   ,  \"στS\" -> 0.000185539060   ,  \"στN\" -> 0.000003670517    |>   , \n\"IDS0468_220530_RAW_cal__sam_\" ->   <|    \"ζ\" -> 0.000000000000   ,  \"τ1\" -> 0.000000000000   ,  \"τS\" -> 0.000000000000   ,  \"τN\" -> 0.000000000000   ,  \"τC\" -> 0.000000000000   ,  \"κ0\" -> 0.000000000000   ,  \"mm1\" -> 0.000000000000   ,  \"mm2\" -> 0.000000000000   ,  \"mm3\" -> 0.000000000000   ,  \"T\" -> 0.820000000000   ,  \"B\" -> 4.000000000000   ,  \"θ\" -> 0.000000000000   ,  \"Reoff\" -> 0.000000000000   ,  \"Imoff\" -> 0.000000000000   ,  \"στ1\" -> 0.000000000000   ,  \"στS\" -> 0.000000000000   ,  \"στN\" -> 0.000000000000    |>   , \n\"IDS0469_220530_RAW_cal__ref_\" ->   <|    \"ζ\" -> 0.021661724597   ,  \"τ1\" -> 0.135376034198   ,  \"τS\" -> 0.027370656195   ,  \"τN\" -> 0.000065416524   ,  \"τC\" -> 0.002262892828   ,  \"κ0\" -> 0.000000007163   ,  \"mm1\" -> 0.000044452306   ,  \"mm2\" -> 0.030162834530   ,  \"mm3\" -> 0.135462025560   ,  \"T\" -> 1.120000000000   ,  \"B\" -> 4.000000000000   ,  \"θ\" -> 0.000000000000   ,  \"Reoff\" -> -775510.204081632196   ,  \"Imoff\" -> 0.000000000000   ,  \"στ1\" -> 0.011862460543   ,  \"στS\" -> 0.000298822899   ,  \"στN\" -> 0.000002245413    |>   , \n\"IDS0469_220530_RAW_cal__sam_\" ->   <|    \"ζ\" -> 0.000000000000   ,  \"τ1\" -> 0.000000000000   ,  \"τS\" -> 0.000000000000   ,  \"τN\" -> 0.000000000000   ,  \"τC\" -> 0.000000000000   ,  \"κ0\" -> 0.000000000000   ,  \"mm1\" -> 0.000000000000   ,  \"mm2\" -> 0.000000000000   ,  \"mm3\" -> 0.000000000000   ,  \"T\" -> 1.120000000000   ,  \"B\" -> 4.000000000000   ,  \"θ\" -> 0.000000000000   ,  \"Reoff\" -> 0.000000000000   ,  \"Imoff\" -> 0.000000000000   ,  \"στ1\" -> 0.000000000000   ,  \"στS\" -> 0.000000000000   ,  \"στN\" -> 0.000000000000    |>   , \n\"IDS0470_220530_RAW_cal__ref_\" ->   <|    \"ζ\" -> 0.015441202200   ,  \"τ1\" -> 0.041977704334   ,  \"τS\" -> 0.036507196019   ,  \"τN\" -> 0.000016236903   ,  \"τC\" -> 0.002199544538   ,  \"κ0\" -> 0.000000012895   ,  \"mm1\" -> 0.000031599194   ,  \"mm2\" -> 0.039021251943   ,  \"mm3\" -> 0.042211796370   ,  \"T\" -> 1.900000000000   ,  \"B\" -> 4.000000000000   ,  \"θ\" -> 0.000000000000   ,  \"Reoff\" -> -265306.122448978945   ,  \"Imoff\" -> 0.000000000000   ,  \"στ1\" -> 0.036878491395   ,  \"στS\" -> 0.000608860312   ,  \"στN\" -> 0.000004645190    |>   , \n\"IDS0470_220530_RAW_cal__sam_\" ->   <|    \"ζ\" -> 0.000000000000   ,  \"τ1\" -> 0.000000000000   ,  \"τS\" -> 0.000000000000   ,  \"τN\" -> 0.000000000000   ,  \"τC\" -> 0.000000000000   ,  \"κ0\" -> 0.000000000000   ,  \"mm1\" -> 0.000000000000   ,  \"mm2\" -> 0.000000000000   ,  \"mm3\" -> 0.000000000000   ,  \"T\" -> 1.900000000000   ,  \"B\" -> 4.000000000000   ,  \"θ\" -> 0.000000000000   ,  \"Reoff\" -> 0.000000000000   ,  \"Imoff\" -> 0.000000000000   ,  \"στ1\" -> 0.000000000000   ,  \"στS\" -> 0.000000000000   ,  \"στN\" -> 0.000000000000    |>   , \n\"IDS0471_220530_RAW_cal__ref_\" ->   <|    \"ζ\" -> 0.014899977348   ,  \"τ1\" -> 0.039852327400   ,  \"τS\" -> 0.012042479771   ,  \"τN\" -> 0.000007668254   ,  \"τC\" -> 0.002248141599   ,  \"κ0\" -> 0.000000015723   ,  \"mm1\" -> 0.000027931492   ,  \"mm2\" -> 0.014437702970   ,  \"mm3\" -> 0.039864529495   ,  \"T\" -> 2.300000000000   ,  \"B\" -> 4.000000000000   ,  \"θ\" -> 0.000000000000   ,  \"Reoff\" -> -183673.469387754798   ,  \"Imoff\" -> 0.000000000000   ,  \"στ1\" -> 0.000774965788   ,  \"στS\" -> 0.000109876194   ,  \"στN\" -> 0.000000141932    |>   , \n\"IDS0471_220530_RAW_cal__sam_\" ->   <|    \"ζ\" -> 0.000000000000   ,  \"τ1\" -> 0.000000000000   ,  \"τS\" -> 0.000000000000   ,  \"τN\" -> 0.000000000000   ,  \"τC\" -> 0.000000000000   ,  \"κ0\" -> 0.000000000000   ,  \"mm1\" -> 0.000000000000   ,  \"mm2\" -> 0.000000000000   ,  \"mm3\" -> 0.000000000000   ,  \"T\" -> 2.300000000000   ,  \"B\" -> 4.000000000000   ,  \"θ\" -> 0.000000000000   ,  \"Reoff\" -> 0.000000000000   ,  \"Imoff\" -> 0.000000000000   ,  \"στ1\" -> 0.000000000000   ,  \"στS\" -> 0.000000000000   ,  \"στN\" -> 0.000000000000    |>   , \n\"IDS0472_220530_RAW_cal__ref_\" ->   <|    \"ζ\" -> 0.016604913016   ,  \"τ1\" -> 0.039295846672   ,  \"τS\" -> 0.009676137271   ,  \"τN\" -> 0.000004030512   ,  \"τC\" -> 0.002212920920   ,  \"κ0\" -> 0.000000022506   ,  \"mm1\" -> 0.000029579758   ,  \"mm2\" -> 0.012018345525   ,  \"mm3\" -> 0.039301748436   ,  \"T\" -> 3.070000000000   ,  \"B\" -> 4.000000000000   ,  \"θ\" -> 0.000000000000   ,  \"Reoff\" -> -183673.469387754798   ,  \"Imoff\" -> 0.000000000000   ,  \"στ1\" -> 0.024245559529   ,  \"στS\" -> 0.008314224018   ,  \"στN\" -> 0.000009266489    |>   , \n\"IDS0472_220530_RAW_cal__sam_\" ->   <|    \"ζ\" -> 0.000000000000   ,  \"τ1\" -> 0.000000000000   ,  
